vi "Create Progress Bar Events.vi"(8 "error in (no error)":errorcluster, 11 "NI_AB_API_Build in":refnum<class "NI_AB_API_Build.lvclass">) -> (0 "error out":errorcluster, 2 "progressBarEvents":T1, 3 "NI_AB_API_Build out":refnum<class "NI_AB_API_Build.lvclass">)   [LabVIEW 2020, in "NI_AB_API_Build.lvclass"]
uses:
  <vilib>/AppBuilder/AB_API/Build/NI_AB_API_Build.lvclass
  <vilib>/AppBuilder/AB_API/common/AB_API ProgressBar_Events.ctl
  <vilib>/AppBuilder/AB_API/common/AB_API ProgressBar_BuildError.ctl
  <vilib>/AppBuilder/AB_API/Build/NI_AB_API_Build.lvclass/NI_AB_API_Build.ctl
  <vilib>/AppBuilder/AB_Classes/Build/AB_Build.lvclass
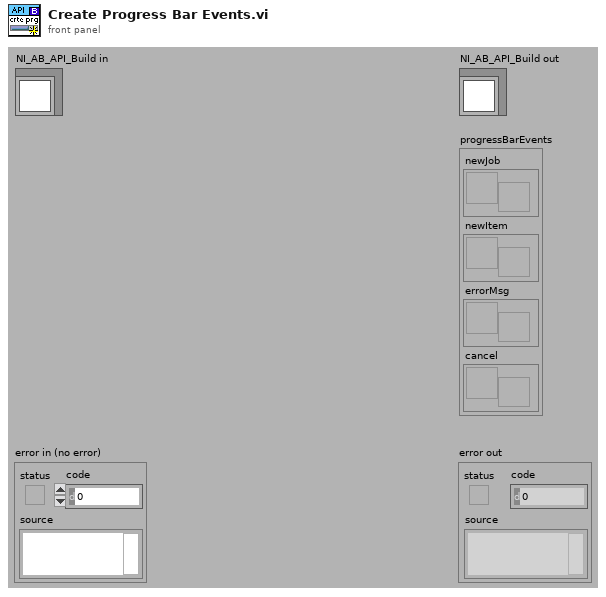
[diagram p1: front panel]
types:
  T1 = typedef "AB_API ProgressBar_Events.ctl" = cluster{"newJob":refnum<user-event>, "newItem":refnum<user-event>, "errorMsg":T2, "cancel":refnum<user-event>}
  T2 = typedef "AB_API ProgressBar_BuildError.ctl" = refnum<user-event>
  T3 = typedef "AB_Build.ctl" = cluster{"buildSpecName":string, "buildSpecDescription":string, "destinations":refnum<class "AB_Destination.lvclass">[], "exclusionOption":T4, "defaultLanguage":string, "supportedLanguages":string[], "excludedDirectories":path[], "buildContext":refnum<vi>, "buildObject":T5, "preview":bool, "programatic":bool, "progressBarEvents":T6, "userLog_Path":path, "preActionID":string, "preAction_Path":path, "postActionID":string, "postAction_Path":path, "eng_checkForBrokenVIs?":bool, "eng_verboseLinkerErrors?":bool, "localDest_Path":path, "targetDest_Path":path, "removeVIObject":u16, "cache":refnum<class "PreviewCache.lvclass">, "use cache":bool, "previewCache_ID":string, "buildCache_ID":string, "eng_TempLocalDest_Path":path, "eng_collectDependencies?":bool, "versionInfo":cluster{"buildVersion":cluster{"major":u16, "minor":u16, "patch":u16, "build":u16}, "autoIncrement":bool}, "eng_enableVIChecksums":bool}
  T4 = typedef "AB_Exclusion_Option.ctl" = cluster{"typedefs":bool, "polymorphicVIs":bool, "unusedLibraryItems":bool, "modifyLibraryFile":bool, "edit-timeDependencies":bool, "inlineVIs":bool, "dependent PPLs":bool, "dependent DLLs":bool}
  T5 = typedef "ItemRef.ctl" = u64
  T6 = typedef "provcom_ProgressBar_Events.ctl" = cluster{"newJob":refnum<user-event>, "newItem":refnum<user-event>, "errorMsg":T7, "cancel":refnum<user-event>}
  T7 = typedef "mxLvBuildError.ctl" = refnum<user-event>
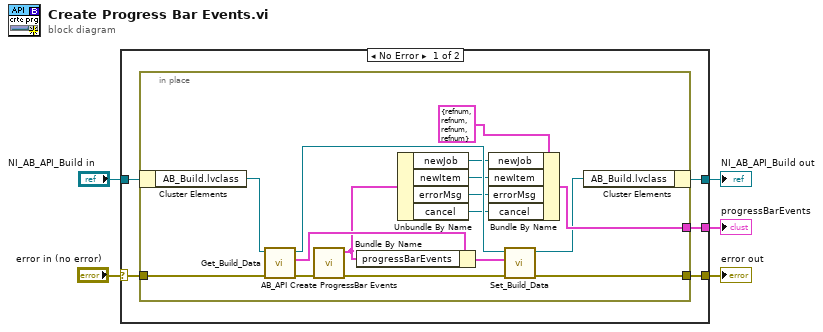
[diagram p0: block diagram]
diagram:
  n1 = case shown="No Error" "error in (no error)" {
    selector: "error in (no error)" -> [w10 w28]
    tunnel: [w9 w28] -> w4
    tunnel: [w6 w27] -> w2
    tunnel: "NI_AB_API_Build in" -> [w7 w27]
    tunnel: [w8 _] -> w1
    frame No Error {
      n2 = in-place {
        in-place-border: w10 -> [w13]
        in-place-border: [w11] -> w9
        in-place-border: [w26] -> w8
        n3 = in-place-cluster #1(w7) -> ("AB_Build.lvclass"=w16:refnum<class "AB_Build.lvclass">)
        n4 = call <vilib>:"Get_Build_Data.vi"("error in (no error)"=w13, "Class in"=w16) -> ("error out"=w14:errorcluster, "data"=w24:T3, "Class out"=w25:refnum<class "AB_Build.lvclass">)  [unwired: 7 in]
        n5 = call <vilib>:"AB_API Create ProgressBar Events.vi"("error in (no error)"=w14) -> ("error out"=w12:errorcluster, "progressBarEvents"=w18:T6)  [unwired: 9 in]
        n6 = Bundle By Name(cluster=w24, "progressBarEvents"=w18) -> (w23:T3)
        n7 = Unbundle By Name(w18) -> ("newJob"=w22:refnum<user-event>, "newItem"=w21:refnum<user-event>, "errorMsg"=w20:T7, "cancel"=w19:refnum<user-event>)
        n8 = Bundle By Name(cluster=T1 {"newJob"=refnum, "newItem"=refnum, "errorMsg"=refnum, "cancel"=refnum} ("progressBarEvents"), "newJob"=w22, "newItem"=w21, "errorMsg"=w20, "cancel"=w19) -> (w26:T1)
        n9 = call <vilib>:"Set_Build_Data.vi"("error in (no error)"=w12, "data"=w23, "Class in"=w25) -> ("error out"=w11:errorcluster, "Class out"=w15:refnum<class "AB_Build.lvclass">)  [unwired: 7 in]
        n10 = in-place-cluster #1("AB_Build.lvclass"=w15) -> (w6:refnum<class "NI_AB_API_Build.lvclass">)
      }
    }
    frame Error {
    }
  }
  "error out" <- w4
  "NI_AB_API_Build out" <- w2
  "progressBarEvents" <- w1
